vi "hex_to_U32.vi"(9 "hex":string) -> (2 "U32":u32)   [LabVIEW 2021]
panel:
  out "unsigned byte array":u8[](array[numeric])
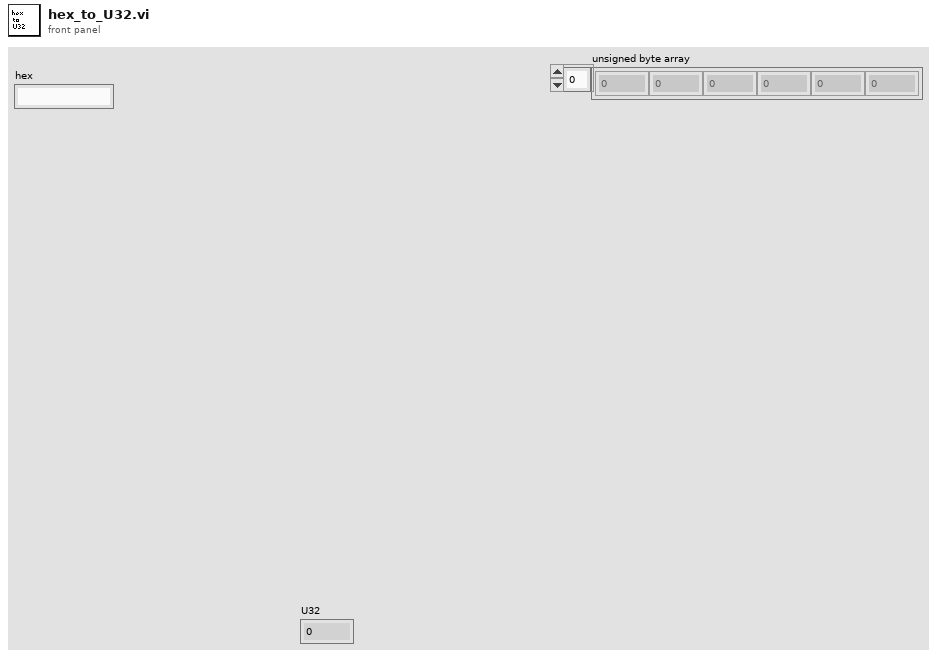
[diagram p1: front panel]
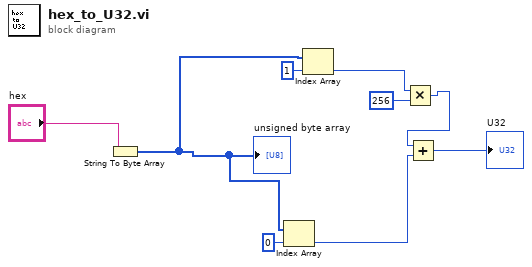
[diagram p0: block diagram]
diagram:
  n1 = String To Byte Array(string="hex") -> (unsigned byte array=w5:u8[])
  "unsigned byte array" <- w5
  n2 = Index Array(array=w5, index=0) -> (element=w4:u8)
  n3 = Index Array(array=w5, index=1) -> (element=w7:u8)
  n4 = Multiply(x=w7, y=u32 256) -> (x*y=w3:u32)
  n5 = Add(x=w3, y=w4) -> (x+y=→"U32":u32)
